vi "Read SystemStatus Event.vi"(8 "error in (no error)":errorcluster, 11 "Engine in":refnum<class "Engine.lvclass">) -> (0 "error out":errorcluster, 2 "SystemStatus Event":refnum<user-event>, 3 "Engine out":refnum<class "Engine.lvclass">)   [LabVIEW 2023, in "Engine.lvlib" / "Engine.lvclass"]
uses:
  Project/Engine.lvclass
  Custom Controls/System Status.ctl
  Project/Engine.lvclass/Engine.ctl
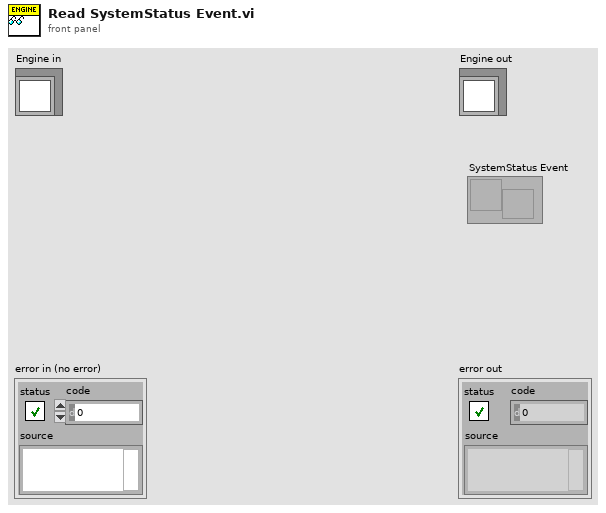
[diagram p1: front panel]
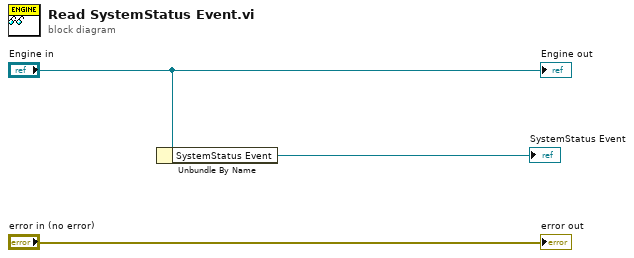
[diagram p0: block diagram]
diagram:
  n1 = Unbundle By Name("Engine in") -> ("SystemStatus Event"=→"SystemStatus Event":refnum<user-event>)
  "error out" <- "error in (no error)"
  "Engine out" <- "Engine in"
